vi "Swerve Motor Back Left old.vi"(0 "Steer motor reference name":string="My Motor RefNum", 1 "Drive motor reference name":string="My Motor RefNum", 2 "Speed command":dbl, 3 "Direction command (deg)":dbl) -> ()   [LabVIEW 2018]
uses:
  <vilib>/Rock Robotics/WPI/ThirdParty/REV Robotics/SPARK MAX/Typedef/Spark MAX Control Type.ctl
  <vilib>/Rock Robotics/WPI/ThirdParty/Phoenix-LabVIEW/Motor Controller/Controls/CTRE_Phoenix_MotorControl_ControlMode.ctl
  <vilib>/Rock Robotics/WPI/ThirdParty/Phoenix-LabVIEW/Motor Controller/Get/CTRE_Phoenix_MotorController_GetAnalogData.vi
  Robot Global Data.vi
panel:
  out "New Posiition 2":dbl
  out "Degres To Travel":dbl
  out "Corrected angle":dbl
  out "Veloicity":dbl
  out "New Posiition":dbl
  out "Back Left Angle":dbl
  out "Position (Raw Sensor Units)":i32
  # "VI inputs"
  # "Intermediate values"
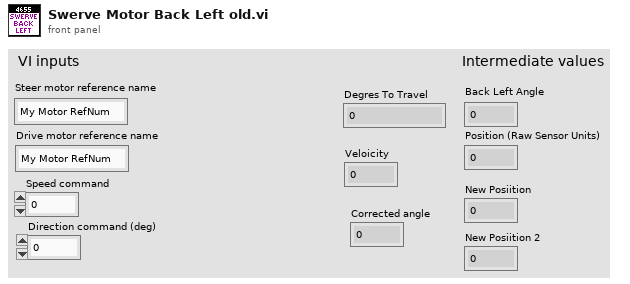
[diagram p1: front panel]
types:
  T1 = typedef "Spark MAX Control Type.ctl" = enum16{"Percent VBus", "Voltage", "Velocity", "Position", "Smart Motion", "Current", "Smart Velocity"}
  T2 = typedef "WPI_MotorControlDeviceRef.ctl" = cluster{"DeviceStatus":errorcluster, "Type":T3, "PWM":cluster{"PWM Channel":T4, "DeadBand":T5}, "CAN":cluster{"Device Number":u8, "SetOutput VI Ref":variant, "GetOutput VI Ref":variant, "Enable VI Ref":variant, "Disable VI Ref":variant, "Data":variant}, "Invert":bool, "DIO PWM":cluster{"PWM \"Enable\" Channel":T4, "DIOChannel":T6, "PWM Rate":dbl}}
  T3 = typedef "WPI_MotorControlType.ctl" = enum16{"PWM", "CAN", "DIO PWM"}
  T4 = typedef "FPGA_DIOPWMChannel.ctl" = enum8{"PWM 0", "PWM 1", "PWM 2", "PWM 3", "PWM 4", "PWM 5", "PWM 6", "PWM 7", "PWM 8", "PWM 9", "PWM MXP 0", "PWM MXP 1", "PWM MXP 2", "PWM MXP 3", "PWM MXP 4", "PWM MXP 5", "PWM MXP 6", "PWM MXP 7", "PWM MXP 8", "PWM MXP 9", "Invalid"}
  T5 = typedef "WPI_PWMDeadband.ctl" = cluster{"Name":string, "maxPositivePwm":i32, "minPositivePwm":i32, "centerPwm":i32, "maxNegativePwm":i32, "minNegativePwm":i32, "angularRange":u16}
  T6 = typedef "FPGA_DIOChannel.ctl" = enum8{"DIO 0", "DIO 1", "DIO 2", "DIO 3", "DIO 4", "DIO 5", "DIO 6", "DIO 7", "DIO 8", "DIO 9", "DIO MXP 0", "DIO MXP 1", "DIO MXP 2", "DIO MXP 3", "DIO MXP 4", "DIO MXP 5", "DIO MXP 6", "DIO MXP 7", "DIO MXP 8", "DIO MXP 9", "DIO MXP 10", "DIO MXP 11", "DIO MXP 12", "DIO MXP 13", "DIO MXP 14", "DIO MXP 15", "SPI Port CS1", "SPI Port CS2", "SPI Port CS3", "SPI Port MISO", "SPI Port MOSI", "Invalid"}
  T7 = typedef "CTRE_Phoenix_MotorControl_ControlMode.ctl" = u16
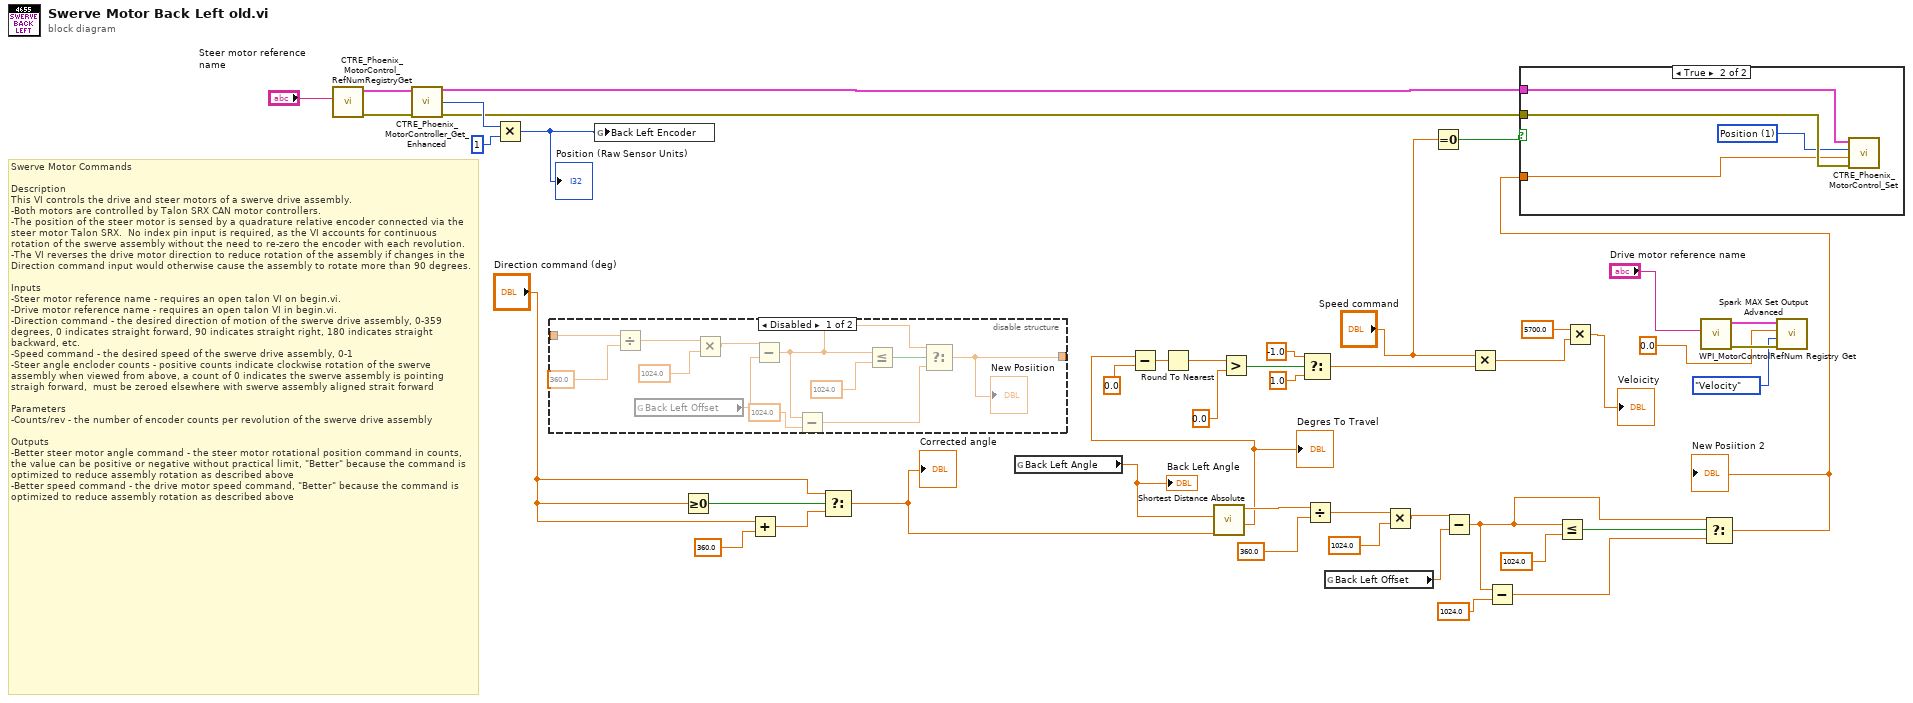
[diagram p0: block diagram]
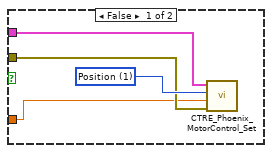
[diagram p3: hidden frame]
diagram:
  # "Swerve Motor Commands\n\nDescription\nThis VI controls the drive and steer motors of a swerve drive assembly.  \n-Both motors are controlled by Talon SRX CAN motor controllers.  \n-The position of the steer motor is sensed by a quadrature relative encoder connected via the steer motor Talon SRX.  No index pin input is required, as the VI accounts for continuous rotation of the swerve assembly without the need to re-zero the encoder with each revolution.\n-The VI reverses the drive motor direction to reduce rotation of the assembly if changes in the Direction command input would otherwise cause the assembly to rotate more than 90 degrees.\n\nInputs\n-Steer motor reference name - requires an open talon VI on begin.vi.\n-Drive motor reference name - requires an open talon VI in begin.vi.\n-Direction command - the desired direction of motion of the swerve drive assembly, 0-359 degrees, 0 indicates straight forward, 90 indicates straight right, 180 indicates straight backward, etc.\n-Speed command - the desired speed of the swerve drive assembly, 0-1\n-Steer angle encloder counts - positive counts indicate clockwise rotation of the swerve assembly when viewed from above, a count of 0 indicates the swerve assembly is pointing straigh forward,  must be zeroed elsewhere with swerve assembly aligned strait forward\n\nParameters\n-Counts/rev - the number of encoder counts per revolution of the swerve drive assembly\n\nOutputs\n-Better steer motor angle command - the steer motor rotational position command in counts, the value can be positive or negative without practical limit, \"Better\" because the command is optimized to reduce assembly rotation as described above\n-Better speed command - the drive motor speed command, \"Better\" because the command is optimized to reduce assembly rotation as described above"
  n1 = call <vilib>:"CTRE_Phoenix_MotorControl_RefNumRegistryGet.vi"("refnum name"="Steer motor reference name") -> ("error out"=w43:errorcluster, "PhoenixMotorControlDevRef"=w44:T2)  [unwired: 9 in]
  n2 = call-poly <vilib>:"CTRE_Phoenix_MotorController_Get_Enhanced.vi"("PhoenixMotorControlDevRef"=w44, "error in"=w43) -> ("PhoenixMotorControlDevRef"=w3:T2, "AnalogInRaw"=w26:i32, "error out"=w2:errorcluster)  [unwired: 9 in, 2 out]
  n3 = Multiply(x=w26, y=1) -> (x*y=w24:i32)
  "Position (Raw Sensor Units)" <- w24
  n4 = disable-structure shown="Disabled" {
    disable-tunnel: [w48 _] -> _
    disable-tunnel: _ -> [w47 _]
    frame Disabled {
      n5 = Divide(x=w47, y=360.0 ("x*y")) -> (x/y=w56:dbl)
      n6 = global read "Robot Global Data.vi" "Back Left Offset"() -> (w53:dbl)
      n7 = Multiply(x=w56, y=1024.0 ("x")) -> (x*y=w54:dbl)
      n8 = Subtract(x=w54, y=w53) -> (x-y=w49:dbl)
      n9 = Subtract(x=w49, y=1024.0 ("x")) -> (x-y=w50:dbl)
      n10 = Less Or Equal?(x=w49, y=1024.0 ("x")) -> (x <= y?=w51:bool)
      n11 = Select(t=w49, s=w51, f=w50) -> (s? t:f=w48:dbl)
      "New Posiition" <- w48
    }
    frame Enabled {
    }
  }
  n12 = global write "Robot Global Data.vi" "Back Left Encoder"(w24) -> ()
  n13 = Greater Or Equal To 0?(x="Direction command (deg)") -> (x >= 0?=w23:bool)
  n14 = Add(x="Direction command (deg)", y=360.0) -> (x+y=w22:dbl)
  n15 = Select(t="Direction command (deg)", s=w23, f=w22) -> (s? t:f=w19:dbl)
  "Corrected angle" <- w19
  n16 = global read "Robot Global Data.vi" "Back Left Angle"() -> (w1:dbl)
  "Back Left Angle" <- w1
  n17 = call "Shortest Distance Absolute.vi"("Current Angle"=w1, "Set Point"=w19) -> ("Better Angle"=w5:dbl, "Degres To Travel"=w4:dbl)  [unwired: 7 in]
  "Degres To Travel" <- w4
  n18 = Subtract(x=w4, y=0.0) -> (x-y=w35:dbl)
  n19 = Round To Nearest(number=w35) -> (nearest integer value=w37:dbl)
  n20 = Greater?(x=w37, y=0.0) -> (0:w34:bool)
  n21 = Select(t=-1.0, s=w34, f=1.0) -> (s? t:f=w32:dbl)
  n22 = Divide(x=w5, y=360.0 ("x*y")) -> (x/y=w15:dbl)
  n23 = global read "Robot Global Data.vi" "Back Left Offset"() -> (w12:dbl)
  n24 = Multiply(x=w15, y=1024.0 ("x")) -> (x*y=w13:dbl)
  n25 = Equal To 0?(x="Speed command") -> (x = 0?=w28:bool)
  n26 = Subtract(x=w13, y=w12) -> (x-y=w8:dbl)
  n27 = Multiply(x="Speed command", y=w32) -> (x*y=w30:dbl)
  n28 = Subtract(x=w8, y=1024.0 ("x")) -> (x-y=w9:dbl)
  n29 = Less Or Equal?(x=w8, y=1024.0 ("x")) -> (x <= y?=w10:bool)
  n30 = Multiply(x=5700.0, y=w30) -> (x*y=→"Veloicity":dbl)
  n31 = call <vilib>:"WPI_MotorControlRefNum Registry Get.vi"("refnum name"="Drive motor reference name") -> ("error out"=w40:errorcluster, "MotorControlDevRef"=w39:T2)  [unwired: 9 in]
  n32 = Select(t=w8, s=w10, f=w9) -> (s? t:f=w6:dbl)
  "New Posiition 2" <- w6
  n33 = case shown="True" w28 {
    tunnel: w3 -> [w60 w65]
    tunnel: w2 -> [w59 w64]
    tunnel: w6 -> [w58 w62]
    frame False {
      w61 = T7 1 items=["PercentOutput"=0, "Position"=1, "Velocity"=2, "Current"=3, "Follower"=5, "MotionProfile"=6, "MotionMagic"=7, "MotionProfileArc"=10, "Disabled"=15] ("Control Mode")
      n34 = call <vilib>:"CTRE_Phoenix_MotorControl_Set.vi"("error in (no error)"=w59, "Output"=w58, "Control Mode"=w61, "PhoenixMotorControlDevRef"=w60) -> ()  [unwired: 6 in, 2 out]
    }
    frame True {
      w63 = T7 1 items=["PercentOutput"=0, "Position"=1, "Velocity"=2, "Current"=3, "Follower"=5, "MotionProfile"=6, "MotionMagic"=7, "MotionProfileArc"=10, "Disabled"=15] ("Control Mode")
      n35 = call <vilib>:"CTRE_Phoenix_MotorControl_Set.vi"("error in (no error)"=w64, "Output"=w62, "Control Mode"=w63, "PhoenixMotorControlDevRef"=w65) -> ()  [unwired: 6 in, 2 out]
    }
  }
  n36 = call <vilib>:"Spark MAX Set Output Advanced.vi"("error in (no error)"=w40, "Control Mode"=Spark_MAX_Control_Type."Velocity", "Setpoint"=0.0, "MotorControlDevRef"=w39) -> ()  [unwired: 6 in, 2 out]
